vi "Write sdaFactory.vi"(10 "sdaFactory":refnum<class "ISDAFactory.lvclass">, 11 "Model in":refnum<class "Model.lvclass">) -> (3 "Model out":refnum<class "Model.lvclass">)   [LabVIEW 2013, in "Model.lvclass"]
uses:
  Model.lvclass
  ISDAFactory/ISDAFactory.lvclass
  Model.lvclass/Model.ctl
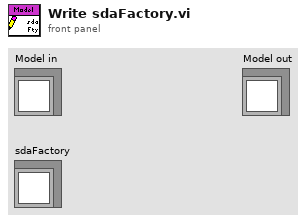
[diagram p1: front panel]
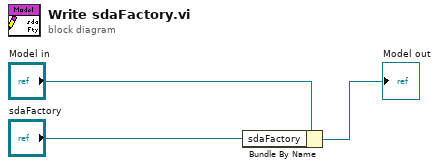
[diagram p0: block diagram]
diagram:
  n1 = Bundle By Name(cluster="Model in", "sdaFactory"="sdaFactory") -> (→"Model out":refnum<class "Model.lvclass">)
